vi "Sweep VBL SET.vi"(6 "Other Fixed Voltage (V)":dbl, 8 "error in (no error)":errorcluster, 10 "Pulse Width (us)":dbl, 11 "Sweep outfile":path) -> (0 "error out":errorcluster, 1 "final current (A)":dbl, 2 "final resistance (ohm)":dbl, 3 "final voltage (V)":dbl)   [LabVIEW 2019]
uses:
  Globals.vi
  <vilib>/Utility/file.llb/Write Delimited Spreadsheet (DBL).vi
panel:
  out "initial resistance (ohm)":dbl format="%#_6p"
  out "VSL (V)":dbl
  out "VBL (V)":dbl
  out "VWL (V)":dbl
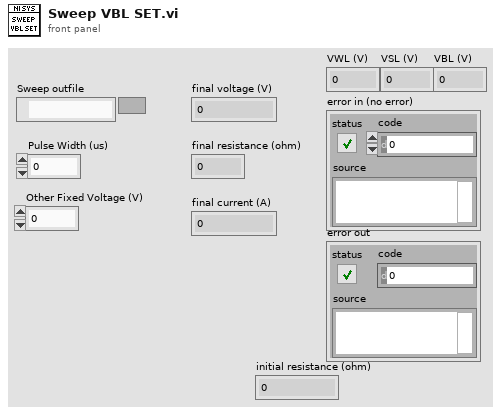
[diagram p1: front panel]
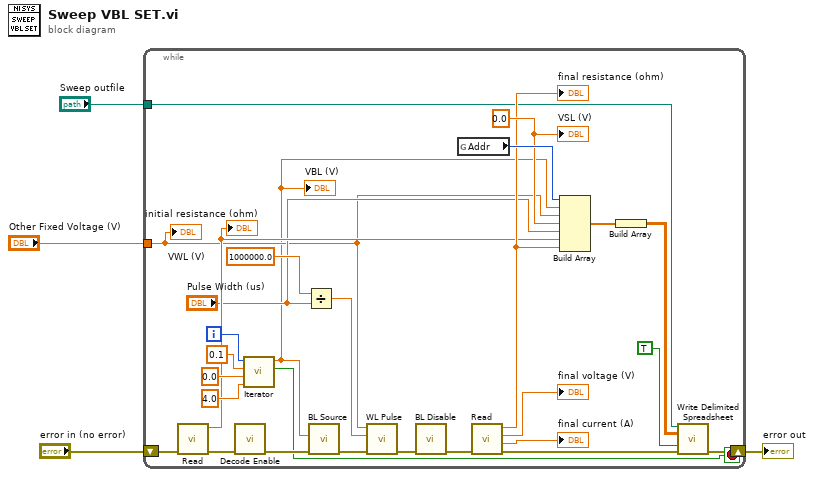
[diagram p0: block diagram]
diagram:
  n1 = while {
    tunnel: "Other Fixed Voltage (V)" -> [w6]
    shift-right: [w8] -> w1
    shift-left: "error in (no error)" -> [w22]
    tunnel: "Sweep outfile" -> [w12]
    i -> [w29]
    stop <- w15 stop-if-true
    w19 = 0.0 ("VSL (V)")
    n2 = call "Read.vi"("error in (no error)"=w22) -> ("error out"=w21:errorcluster, "resistance (ohm)"=w14:dbl)  [unwired: 7 in, 2 out]
    "initial resistance (ohm)" <- w14
    n3 = call "Decode Enable.vi"("error in (no error)"=w21) -> ("error out"=w28:errorcluster)  [unwired: 10 in]
    n4 = call "Iterator.vi"("Final Value"=4.0, "Initial Value"=0.0, "Step"=0.1, "i"=w29) -> ("End Loop"=w15:bool, "Current Value"=w5:dbl)  [unwired: 6 in]
    "VBL (V)" <- w5
    n5 = Divide(x=1000000.0 ("Sample Rate"), y="Pulse Width (us)") -> (x/y=w24:dbl)
    n6 = call "BL Source.vi"("error in (no error)"=w28, "voltage level (V)"=w5) -> ("error out"=w26:errorcluster)  [unwired: 9 in]
    n7 = call "WL Pulse.vi"("error in (no error)"=w26, "Sample Rate"=w24, "VWL (V)"=w6) -> ("error out"=w27:errorcluster)  [unwired: 8 in]
    n8 = call "BL Disable.vi"("error in (no error)"=w27) -> ("error out"=w25:errorcluster)  [unwired: 10 in]
    n9 = global read "Globals.vi" "Addr"() -> (w20:u16)
    n10 = call "Read.vi"("error in (no error)"=w25) -> ("error out"=w11:errorcluster, "current (A)"=→"final current (A)":dbl, "read voltage (V)"=→"final voltage (V)":dbl, "resistance (ohm)"=w16:dbl)  [unwired: 7 in]
    "final resistance (ohm)" <- w16
    n11 = Build Array(w20, w5, w6, w19, "Pulse Width (us)", w14, w16) -> (w10:dbl[])
    n12 = Build Array(w10) -> (w9:dbl[][])
    n13 = call-poly <vilib>:"Write Delimited Spreadsheet.vi"("file path (dialog if empty)"=w12, "2D data"=w9, "append to file? (new file:F)"=TRUE, "error in (no error)"=w11) -> ("error out"=w8:errorcluster)  [unwired: 10 in, 1 out]
    "VWL (V)" <- w6
    "VSL (V)" <- w19
  }
  "error out" <- w1
